vi "main.vi"() -> ()   [LabVIEW 2016]
panel:
  out "Velocities":cluster{dbl, dbl, dbl}(graph)
  out "Facing":dynamicdata(graph)
  out "Startup Status":u8
  in  "?":bool
  # "Connect the IMU to the B pins on the myRIO"
  # "104 means good to go"
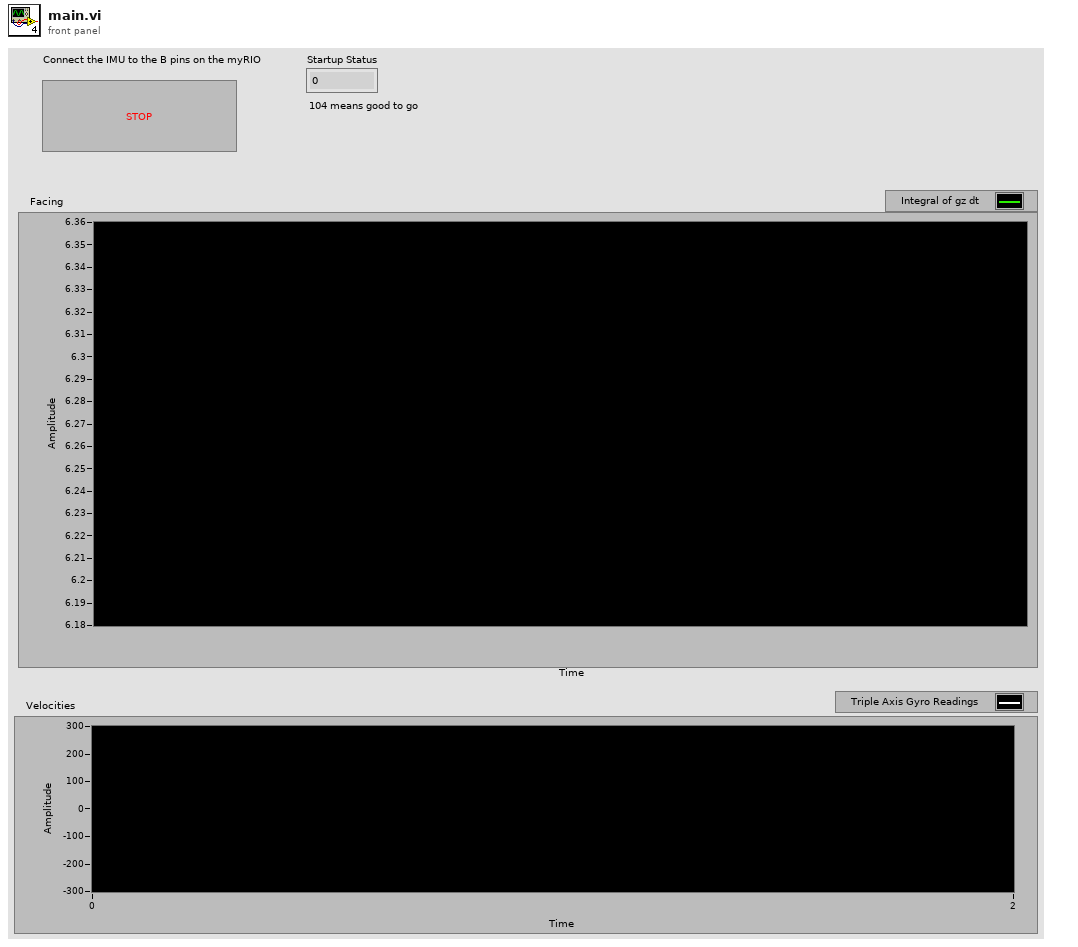
[diagram p1: front panel]
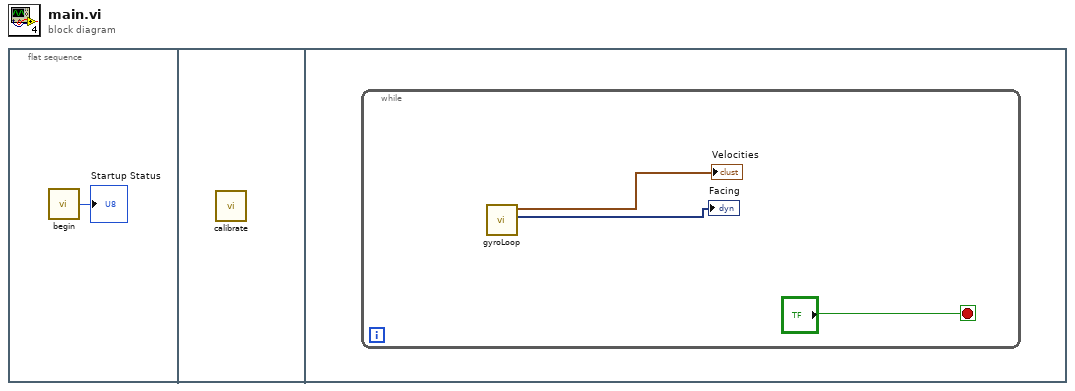
[diagram p0: block diagram]
diagram:
  n1 = flat-sequence {
    frame #0 {
      n2 = call "begin.vi"() -> ("xgTest"=→"Startup Status":u8)  [unwired: 1 in]
    }
    frame #1 {
      n3 = call "calibrate.vi"() -> ()  [unwired: 12 in]
    }
    frame #2 {
      n4 = while {
        stop <- "?" stop-if-true
        n5 = call "gyroLoop.vi"() -> ("Facing"=→"Facing":dynamicdata, "Velocities"=→"Velocities":cluster{dbl, dbl, dbl})  [unwired: 10 in]
      }
    }
  }
